vi "Utility - Configuration File Generator.vi"() -> ()   [LabVIEW 2018]
uses:
  controls/TDMS Properties.ctl
  controls/Acquisition and Logging Configuration.ctl
  <vilib>/LabVIEW Targets/FPGA/cRIO/shared/nicrio_ModuleControls/nicrio_cRIO-9237_DataRatesRing.ctl
  <vilib>/LabVIEW Targets/FPGA/cRIO/shared/nicrio_ModuleControls/nicrio_cRIO-9237_ExcitationVoltageRing.ctl
  <vilib>/Utility/xml.llb/Write to XML File(string).vi
panel:
  in  "Data File Name 9222_9049":string="cRIO_Data_9222_9049"
  in  "Number of Channels 9222_9049":i32=28
  in  "Channel Names 9222_9049":string[](array[string])=["Mod1/ai0/PP_0_10_F", "Mod1/ai1/PP_0_10_B", "Mod1/ai2/PP_0_20", "Mod1/ai3/PP_0_30", "Mod2/ai0/PP_0_50", "Mod2/ai1/PP_120_10_F", "Mod2/ai2/PP_120_10_B", "Mod2/ai3/PP_120_20", "Mod3/ai0/PP_120_30", "Mod3/ai1/PP_120_50", "Mod3/ai2/PP_240_10_F", "Mod3/ai3/PP_240_10_B", "Mod4/ai0/PP_240_20", "Mod4/ai1/PP_240_30", "Mod4/ai2/PP_240_50", "Mod4/ai3/ACCEL_", "Mod5/ai0/ACCEL_", "Mod5/ai1/ACCEL_", "Mod5/ai2/ACCEL_A", "Mod5/ai3/PP_A_1", "Mod6/ai0/PP_A_2", "Mod6/ai1/PP_A_3", "Mod6/ai2/PP_A_4", "Mod6/ai3/PP_A_5", "Mod7/ai0/PP_A_6", "Mod7/ai1/AX200", "Mod7/ai2/FAR_FIELD_CAM", "Mod7/ai3/SPECTRAL_ANALYZER"]
  in  "TDMS Properties 9237":T1[](array[typedef])=[{"Name"="J_Schwartz", "Value"="BEi"}, {"Name"="Author", "Value"="[DeveloperName]"}, {"Name"="Operator", "Value"="[OperatorName]"}, {"Name"="TestSystem", "Value"="[SystemName]"}, {"Name"="Site", "Value"="[Location]"}, {"Name"="Line", "Value"="[Line]"}, {"Name"="Machine", "Value"="[MachineName]"}, {"Name"="Description", "Value"="[Description]"}]
  in  "Data File Name 9237":string="cRIO_Data_9237"
  in  "Excitation Voltage":T2 items=["2.5 Volts", "3.3 Volts", "5.0 Volts", "10.0 Volts", "External Excitation"]
  in  "Channel Names 9222_9039":string[](array[string])=["Mod1/ai0/PP_0_10_F", "Mod1/ai1/PP_0_10_B", "Mod1/ai2/PP_0_20", "Mod1/ai3/PP_0_30", "Mod2/ai0/PP_0_50", "Mod2/ai1/PP_120_10_F", "Mod2/ai2/PP_120_10_B", "Mod2/ai3/PP_120_20", "Mod3/ai0/PP_120_30", "Mod3/ai1/PP_120_50", "Mod3/ai2/PP_240_10_F", "Mod3/ai3/PP_240_10_B", "Mod4/ai0/PP_240_20", "Mod4/ai1/PP_240_30", "Mod4/ai2/PP_240_50", "Mod4/ai3/ACCEL_", "Mod5/ai0/ACCEL_", "Mod5/ai1/ACCEL_", "Mod5/ai2/ACCEL_A", "Mod5/ai3/PP_A_1", "Mod6/ai0/PP_A_2", "Mod6/ai1/PP_A_3", "Mod6/ai2/PP_A_4", "Mod6/ai3/PP_A_5", "Mod7/ai0/PP_A_6", "Mod7/ai1/AX200", "Mod7/ai2/FAR_FIELD_CAM", "Mod7/ai3/SPECTRAL_ANALYZER"]
  in  "Sample Time  9222 [microS]":i32=10
  in  "Samples per Read 9222":i32=10000
  in  "Number of Channels 9222_9039":i32=28
  in  "Data Rate":T3=1 items=["50.000 kS/s (NI 9237)"=1, "25.000 kS/s (NI 9237)"=2, "16.667 kS/s (NI 9237)"=3, "12.500 kS/s (NI 9237)"=4, "10.000 kS/s (NI 9237)"=5, "8.333 kS/s (NI 9237)"=6, "7.143 kS/s (NI 9237)"=7, "6.250 kS/s (NI 9237)"=8, "5.556 kS/s (NI 9237)"=9, "5.000 kS/s (NI 9237)"=10, "4.545 kS/s (NI 9237)"=11, "4.167 kS/s (NI 9237)"=12, "3.846 kS/s (NI 9237)"=13, "3.571 kS/s (NI 9237)"=14, "3.333 kS/s (NI 9237)"=15, "3.125 kS/s (NI 9237)"=16, "2.941 kS/s (NI 9237)"=17, "2.778 kS/s (NI 9237)"=18, "2.632 kS/s (NI 9237)"=19, "2.500 kS/s (NI 9237)"=20, "2.381 kS/s (NI 9237)"=21, "2.273 kS/s (NI 9237)"=22, "2.174 kS/s (NI 9237)"=23, "2.083 kS/s (NI 9237)"=24, "2.000 kS/s (NI 9237)"=25, "1.923 kS/s (NI 9237)"=26, "1.852 kS/s (NI 9237)"=27, "1.786 kS/s (NI 9237)"=28, "1.724 kS/s (NI 9237)"=29, "1.667 kS/s (NI 9237)"=30, "1.613 kS/s (NI 9237)"=31]
  in  "TDMS Properties":T1[](array[typedef])=[{"Name"="Company ", "Value"="BEi"}, {"Name"="Author", "Value"="Jairus Schwartz"}, {"Name"="Operator", "Value"="Jairus Schwartz"}, {"Name"="TestSystem", "Value"="MUCTA"}, {"Name"="Site", "Value"="Test Area 2"}, {"Name"="", "Value"=""}, {"Name"="", "Value"=""}, {"Name"="", "Value"=""}]
  in  "Trigger - Time (Minute)":i32=30
  in  "Trigger - Channel":i32
  in  "Trigger - RMS Value":dbl=1.8
  in  "Channel Names":string[](array[string])=["Mod1/ai0", "Mod1/ai1", "Mod1/ai2", "Mod1/ai3", "Mod2/ai0", "Mod2/ai1", "Mod2/ai2", "Mod2/ai3"]
  in  "Channel Scale Array [Not needed]":fxp<+,24,12>[](array[numeric])=[1.0, 1.0, 1.0, 1.0]
  in  "Number of Channels":i32=8
  in  "Data File Name 9039":string="cRIO_Data_9222_9039"
  in  "Number of Reads to Save":i32=30
  in  "Samples per Read":i32=10000
  # "Instructions: Populate the controls below with desired values, then run the VI to generate a 'Config.xml' file in the root folder of your project.  \n\nNote:  Once you have generated the Config.xml file, you will need to copy it to the root folder of your RT Target."
  # "9237 Acquisition 9049"
  # "9237 Channels 9049"
  # "9237 Logging"
  # "9222 Acquisition"
  # "9222 Channels 9039"
  # "9222 Logging"
  # "Trigger AND Acquistion Time"
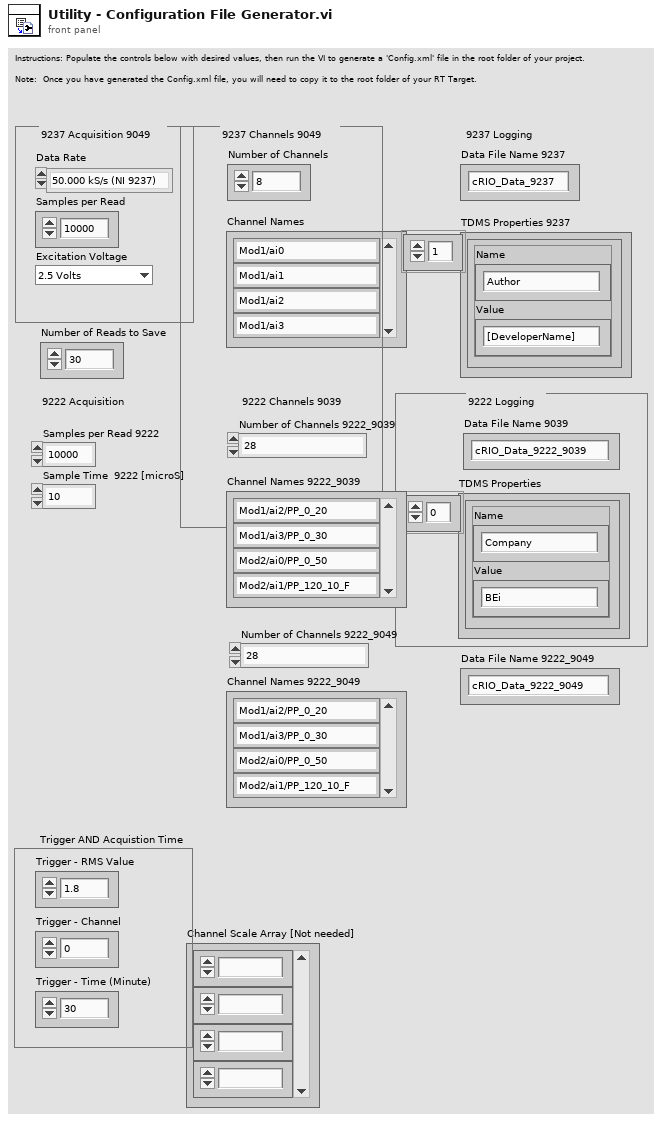
[diagram p1: front panel]
types:
  T1 = typedef "TDMS Properties.ctl" = cluster{"Name":string, "Value":string}
  T2 = typedef "nicrio_cRIO-9237_ExcitationVoltageRing.ctl" = u8
  T3 = typedef "nicrio_cRIO-9237_DataRatesRing.ctl" = u8
  T4 = typedef "Acquisition and Logging Configuration.ctl" = cluster{"Samples per Read":i32, "Number of Reads to Save":i32, "Data File Name 9222_9039":string, "TDMS Properties 9222":T1[], "Number of Channels 9237":i32, "Channel Scale Array":fxp<+,24,12>[], "Channel Names":string[], "Trigger - RMS Value":dbl, "Trigger - Channel":i32, "Trigger - Time (Minute)":i32, "Data Rate 9237":T3, "Number of Channels 9222_9039":i32, "Samples per Read 9222":i32, "Data Rate 9222":i32, "Channel Names 9222_9039":string[], "TDMS Properties 9237":T1[], "Data File Name 9237":string, "Excitation Voltage":T2, "Data File Name 9222_9049_9149":string, "Number of Channels 9222_9049_9149":i32, "Channel Names 9222_9049_9149":string[], "Data File Name 9222_9049_MAIN":string, "Number of Channels 9222_9049_MAIN":i32, "Channel Names 9222_9049_MAIN":string[]}
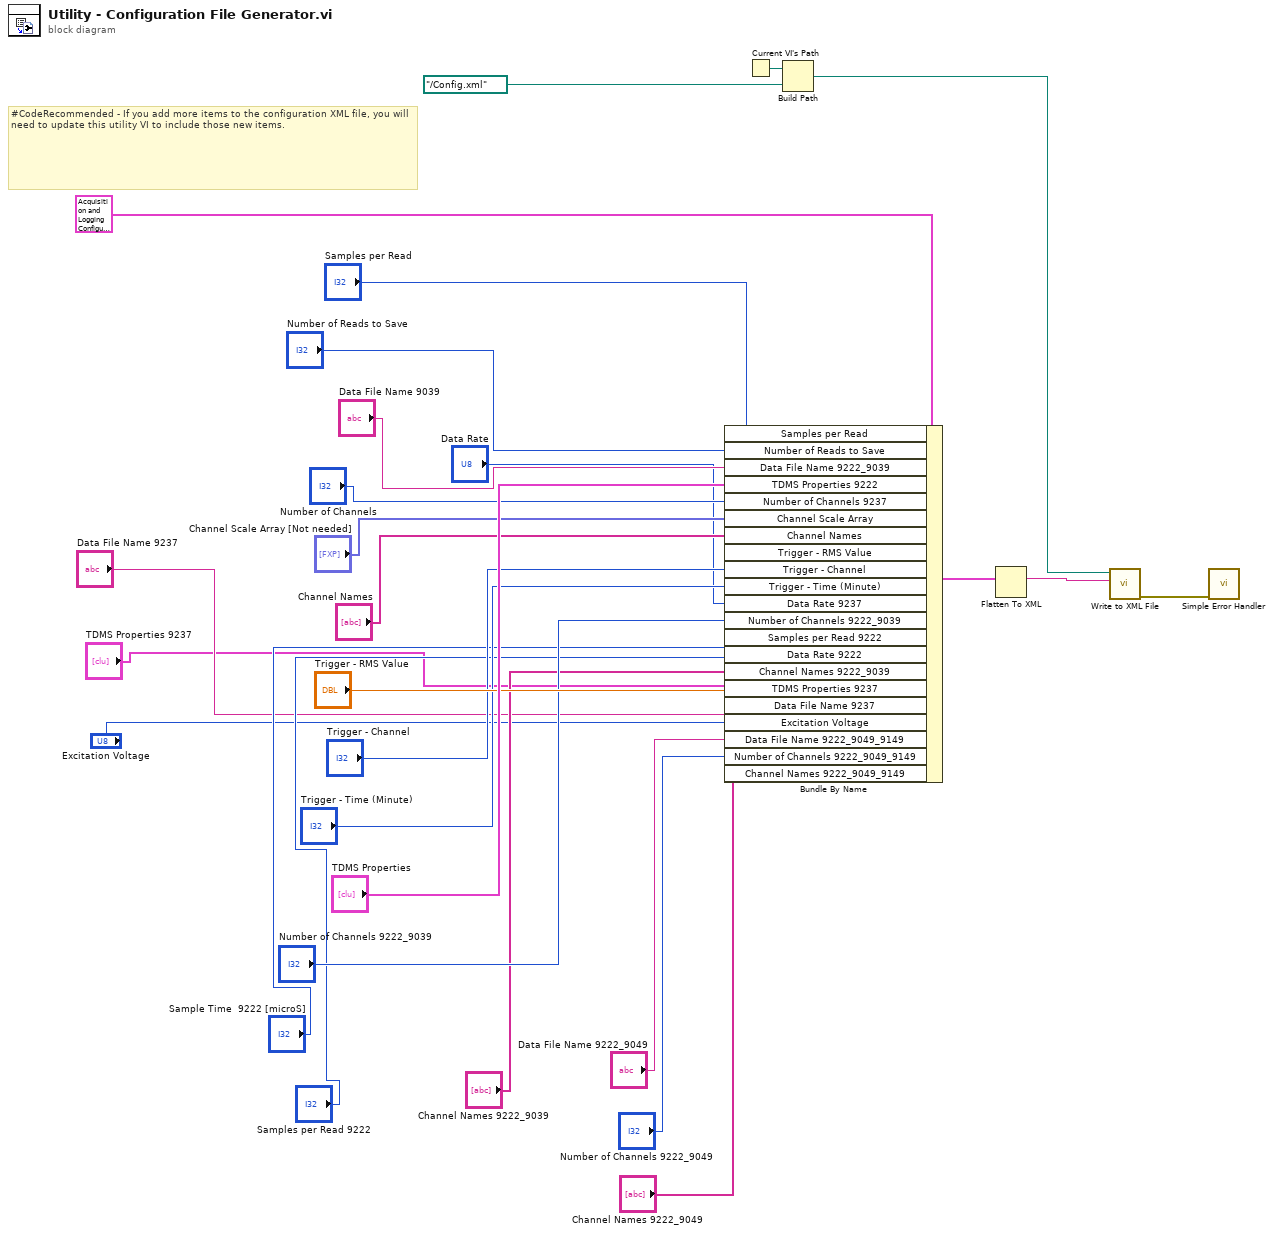
[diagram p0: block diagram]
diagram:
  # "#CodeRecommended - If you add more items to the configuration XML file, you will need to update this utility VI to include those new items."
  n1 = Bundle By Name(cluster=T4 {"Samples per Read"=0, "Number of Reads to Save"=0, "Data File Name 9222_9039"="", "TDMS Properties 9222"=[], "Number of Channels 9237"=0, "Channel Scale Array"=[0.0, 0.0, 0.0, 0.0], "Channel Names"=[], "Trigger - RMS Value"=0.0, "Trigger - Channel"=0, "Trigger - Time (Minute)"=0, "Data Rate 9237"=1, "Number of Channels 9222_9039"=4, "Samples per Read 9222"=0, "Data Rate 9222"=0, "Channel Names 9222_9039"=["Mod1/ai0", "Mod1/ai1", "Mod1/ai2", "Mod1/ai3"], "TDMS Properties 9237"=[], "Data File Name 9237"="", "Excitation Voltage"=0, "Data File Name 9222_9049_9149"="cRIO_Data_9222_9049", "Number of Channels 9222_9049_9149"=28, "Channel Names 9222_9049_9149"=["Mod1/ai0/PP_0_10_F", "Mod1/ai1/PP_0_10_B", "Mod1/ai2/PP_0_20", "Mod1/ai3/PP_0_30", "Mod2/ai0/PP_0_50", "Mod2/ai1/PP_120_10_F", "Mod2/ai2/PP_120_10_B", "Mod2/ai3/PP_120_20", "Mod3/ai0/PP_120_30", "Mod3/ai1/PP_120_50", "Mod3/ai2/PP_240_10_F", "Mod3/ai3/PP_240_10_B", "Mod4/ai0/PP_240_20", "Mod4/ai1/PP_240_30", "Mod4/ai2/PP_240_50", "Mod4/ai3/ACCEL_", "Mod5/ai0/ACCEL_", "Mod5/ai1/ACCEL_", "Mod5/ai2/ACCEL_A", "Mod5/ai3/PP_A_1", "Mod6/ai0/PP_A_2", "Mod6/ai1/PP_A_3", "Mod6/ai2/PP_A_4", "Mod6/ai3/PP_A_5", "Mod7/ai0/PP_A_6", "Mod7/ai1/AX200", "Mod7/ai2/FAR_FIELD_CAM", "Mod7/ai3/SPECTRAL_ANALYZER"], "Data File Name 9222_9049_MAIN"="cRIO_Data_9222_9049", "Number of Channels 9222_9049_MAIN"=28, "Channel Names 9222_9049_MAIN"=["Mod1/ai0/PP_0_10_F", "Mod1/ai1/PP_0_10_B", "Mod1/ai2/PP_0_20", "Mod1/ai3/PP_0_30", "Mod2/ai0/PP_0_50", "Mod2/ai1/PP_120_10_F", "Mod2/ai2/PP_120_10_B", "Mod2/ai3/PP_120_20", "Mod3/ai0/PP_120_30", "Mod3/ai1/PP_120_50", "Mod3/ai2/PP_240_10_F", "Mod3/ai3/PP_240_10_B", "Mod4/ai0/PP_240_20", "Mod4/ai1/PP_240_30", "Mod4/ai2/PP_240_50", "Mod4/ai3/ACCEL_", "Mod5/ai0/ACCEL_", "Mod5/ai1/ACCEL_", "Mod5/ai2/ACCEL_A", "Mod5/ai3/PP_A_1", "Mod6/ai0/PP_A_2", "Mod6/ai1/PP_A_3", "Mod6/ai2/PP_A_4", "Mod6/ai3/PP_A_5", "Mod7/ai0/PP_A_6", "Mod7/ai1/AX200", "Mod7/ai2/FAR_FIELD_CAM", "Mod7/ai3/SPECTRAL_ANALYZER"]} ("Acquisition and Logging Configuration"), "Samples per Read"="Samples per Read", "Number of Reads to Save"="Number of Reads to Save", "Data File Name 9222_9039"="Data File Name 9039", "TDMS Properties 9222"="TDMS Properties", "Number of Channels 9237"="Number of Channels", "Channel Scale Array"="Channel Scale Array [Not needed]", "Channel Names"="Channel Names", "Trigger - RMS Value"="Trigger - RMS Value", "Trigger - Channel"="Trigger - Channel", "Trigger - Time (Minute)"="Trigger - Time (Minute)", "Data Rate 9237"="Data Rate", "Number of Channels 9222_9039"="Number of Channels 9222_9039", "Samples per Read 9222"="Samples per Read 9222", "Data Rate 9222"="Sample Time  9222 [microS]", "Channel Names 9222_9039"="Channel Names 9222_9039", "TDMS Properties 9237"="TDMS Properties 9237", "Data File Name 9237"="Data File Name 9237", "Excitation Voltage"="Excitation Voltage", "Data File Name 9222_9049_9149"="Data File Name 9222_9049", "Number of Channels 9222_9049_9149"="Number of Channels 9222_9049", "Channel Names 9222_9049_9149"="Channel Names 9222_9049") -> (w8:T4)
  n2 = Current VI's Path() -> (path=w27:path)
  n3 = Build Path(base path=w27, name or relative path=path "../Config.xml") -> (appended path=w25:path)
  n4 = Flatten To XML(anything=w8) -> (xml string=w28:string)
  n5 = call-poly <vilib>:"Write to XML File.vi"("XML Input"=w28, "XML File Path"=w25) -> ("error out"=w24:errorcluster)  [unwired: 7 in, 2 out]
  n6 = call <vilib>:"Simple Error Handler.vi"("error in (no error)"=w24) -> ()  [unwired: 4 in, 5 out]
